vi "Load Device Configs.vi"(8 "error in (no error)":errorcluster, 10 "Device Configs":T1[](array[typedef]), 11 "HAL Manager in":refnum<class "HAL Manager.lvclass">) -> (0 "error out":errorcluster, 3 "HAL Manager out":refnum<class "HAL Manager.lvclass">)   [LabVIEW 2020, in "HAL.lvlib" / "HAL Manager.lvclass"]
uses:
  HAL Manager.lvclass
  Device Config.ctl
  Device/Device.lvclass
  Device/Config Item.ctl
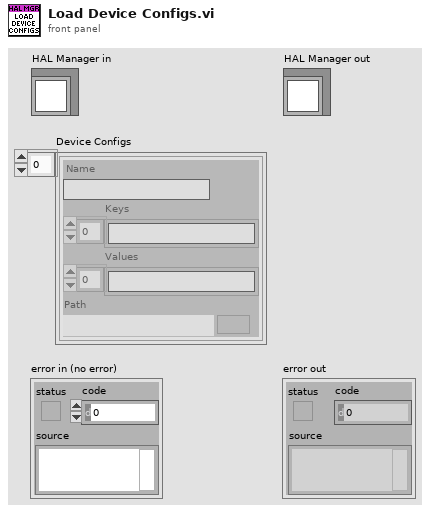
[diagram p1: front panel]
types:
  T1 = typedef "HAL.lvlib/HAL Manager.lvclass/Device Config.ctl" = cluster{"Name":string, "Keys":string[], "Values":string[], "Path":path}
  T2 = typedef "HAL.lvlib/Device.lvclass/Config Item.ctl" = cluster{"Key":string, "Value":string}
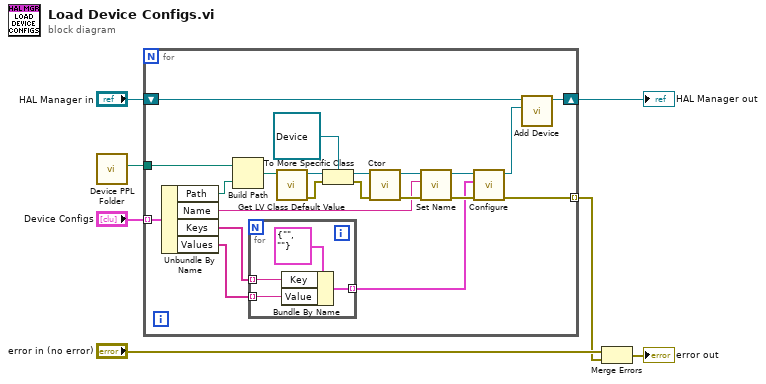
[diagram p0: block diagram]
diagram:
  n1 = call "Device PPL Folder.vi"() -> ("vi path"=w1:path)  [unwired: 8 in, 3 out]
  n2 = for {
    shift-right: [w8] -> w4
    shift-left: "HAL Manager in" -> [w10]
    tunnel: w1 -> [w25]
    tunnel: "Device Configs" -> [w26] mode=indexing
    tunnel: [w11] -> w2 mode=indexing
    n3 = Unbundle By Name(w26) -> ("Path"=w24:path, "Name"=w16:string, "Keys"=w14:string[], "Values"=w13:string[])
    n4 = Build Path(base path=w25, name or relative path=w24) -> (appended path=w23:path)
    n5 = for {
      tunnel: w14 -> [w31] mode=indexing
      tunnel: w13 -> [w30] mode=indexing
      tunnel: [w29] -> w12 mode=indexing
      n6 = Bundle By Name(cluster=T2 {"Key"="", "Value"=""} ("Config Item"), "Key"=w31, "Value"=w30) -> (w29:T2)
    }
    n7 = call <vilib>:"Get LV Class Default Value.vi"("class path"=w23) -> ("error out"=w19:errorcluster, "object"=w22:refnum<class>)  [unwired: 9 in]
    n8 = To More Specific Class(target class=refnum<class "Device.lvclass"> refnum ("HAL.lvlib:Device.lvclass"), reference=w22, error in=w19) -> (specific class reference=w20:refnum<class "Device.lvclass">, error out=w18:errorcluster)
    n9 = call "Ctor.vi"("error in (no error)"=w18, "Device in"=w20) -> ("error out"=w27:errorcluster, "Device out"=w17:refnum<class "Device.lvclass">)  [unwired: 8 in]
    n10 = call "Set Name.vi"("error in (no error)"=w27, "Name"=w16, "Device in"=w17) -> ("error out"=w28:errorcluster, "Device out"=w15:refnum<class "Device.lvclass">)  [unwired: 7 in]
    n11 = call "Configure.vi"("error in (no error)"=w28, "Config"=w12, "Device in"=w15) -> ("error out"=w11:errorcluster, "Device out"=w9:refnum<class "Device.lvclass">)  [unwired: 7 in]
    n12 = call "Add Device.vi"("Device Model"=w9, "HAL Manager in"=w10) -> ("HAL Manager out"=w8:refnum<class "HAL Manager.lvclass">)  [unwired: 7 in, 2 out]
  }
  "HAL Manager out" <- w4
  n13 = Merge Errors("error in (no error)", w2) -> (→"error out":errorcluster)
